vi "UDP Sender.vi"() -> ()   [LabVIEW 2020]
panel:
  in  "stop":bool
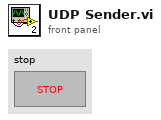
[diagram p1: front panel]
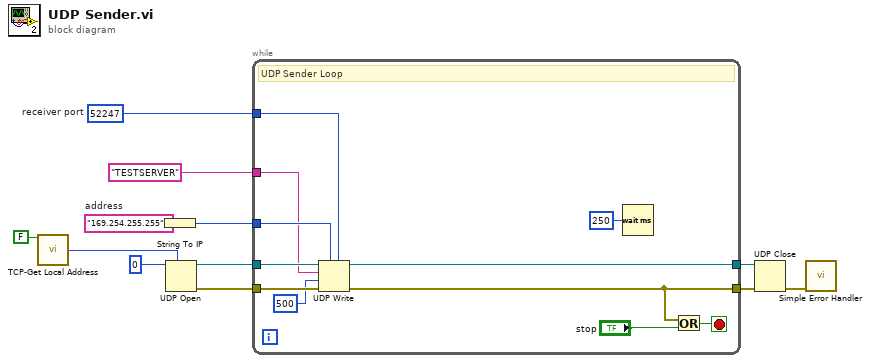
[diagram p0: block diagram]
diagram:
  w6 = u16 52247  # receiver port
  w10 = "169.254.255.255"  # address
  n1 = call "TCP-Get Local Address.vi"("LAN first"=FALSE) -> ("net address"=w1:u32)  [unwired: 13 in, 1 out]
  n2 = String To IP(1:w10) -> (0:w4:u32)
  n3 = UDP Open(7:w1, 11:u16 0 ("port")) -> (port=w8:refnum<k16>, 0:w7:errorcluster)  [unwired: 3 in, 1 out]
  n4 = while {
    tunnel: [w14] -> w11
    tunnel: w8 -> [w23]
    tunnel: w7 -> [w22]
    tunnel: [w15] -> w12
    tunnel: w4 -> [w20]
    tunnel: w6 -> [w16]
    tunnel: "TESTSERVER" -> [w18]
    stop <- w21 stop-if-true
    # "UDP Sender Loop"
    n5 = UDP Write(address=w20, port or service name=w16, connection ID=w23, data in=w18, 8:w22, 9:500 ("timeout ms (25000)")) -> (error out=w14:errorcluster, 3:w15:refnum<k16>)
    n6 = Wait (ms)(milliseconds to wait=u32 250) -> ()  [unwired: 1 out]
    n7 = Or(x=w14, y="stop") -> (x .or. y?=w21:bool)
  }
  n8 = UDP Close(connection ID=w12, 8:w11) -> (error out=w9:errorcluster)  [unwired: 1 out]
  n9 = call <vilib>:"Simple Error Handler.vi"("error in (no error)"=w9) -> ()  [unwired: 4 in, 5 out]
